vi "Start.vi"(8 "error in":errorcluster, 11 "DAQmx Base CFG in":refnum<class "DAQmx Base CFG.lvclass">) -> (0 "error out":errorcluster, 3 "DAQmx Base CFG out":refnum<class "DAQmx Base CFG.lvclass">)   [LabVIEW 2023, in "DAQmx Base CFG.lvclass"]
uses:
  DAQmx Base CFG.lvclass
  Configurations/CFG Base/CFG Base.lvclass/CFG Base.ctl
  DAQmx Base CFG.lvclass/DAQmx Base CFG.ctl
  Configurations/CFG Base/CFG Base.lvclass
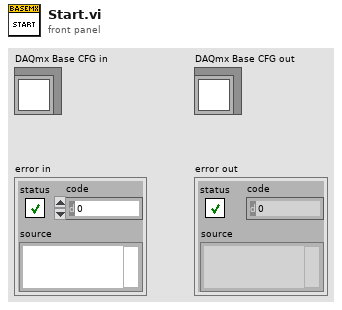
[diagram p1: front panel]
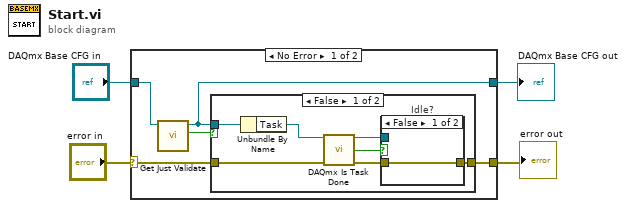
[diagram p0: block diagram]
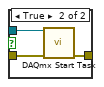
[diagram p2: hidden frame]
diagram:
  n1 = case shown="No Error" "error in" {
    selector: "error in" -> [w7 w23]
    tunnel: "DAQmx Base CFG in" -> [w8 w22]
    tunnel: [w6 w22] -> w1
    tunnel: [w9 w23] -> w2
    frame No Error {
      n2 = call "Get Just Validate.vi"("CFG Base in"=w8) -> ("Just Validate"=w5:bool, "CFG Base out"=w6:refnum<class "DAQmx Base CFG.lvclass">)  [unwired: 9 in]
      n3 = case shown="False" w5 {
        tunnel: [w16 w21] -> w9
        tunnel: w7 -> [w12 w21]
        tunnel: w6 -> [w11 _]
        frame False {
          n4 = Unbundle By Name(w11) -> ("Task"=w10:refnum<k21>)
          n5 = call <vilib>:"DAQmx Is Task Done.vi"("task/channels in"=w10, "error in"=w12) -> ("task out"=w14:refnum<k21>, "task done?"=w13:bool, "error out"=w15:errorcluster)  [unwired: 11 in]
          n6 = case "Idle?" shown="False" w13 {
            tunnel: [w17 w20] -> w16
            tunnel: w15 -> [w17 w19]
            tunnel: w14 -> [_ w18]
            frame False {
            }
            frame True {
              n7 = call <vilib>:"DAQmx Start Task.vi"("task/channels in"=w18, "error in"=w19) -> ("error out"=w20:errorcluster)  [unwired: 12 in, 1 out]
            }
          }
        }
        frame True {
        }
      }
    }
    frame Error {
    }
  }
  "error out" <- w2
  "DAQmx Base CFG out" <- w1
